vi "Demo Multiple Std Dev Calcs.vi"() -> ()   [LabVIEW 2014, in "Exponential Fit Library.lvlib" / "Fit Exponential.lvclass"]
doc: "This is a simle demonstration of the capabilities of the exponential fit class."
uses:
  Fit Exponential.lvclass
panel:
  out "x-y":u32
  out "XY Graph":cluster{"ChunkSize":i32[], "StdDevOut":dbl[]}(graph)
  in  "ChunkSize":i32[](array[numeric])
  in  "# taus":i32
  in  "tau":dbl=60.0
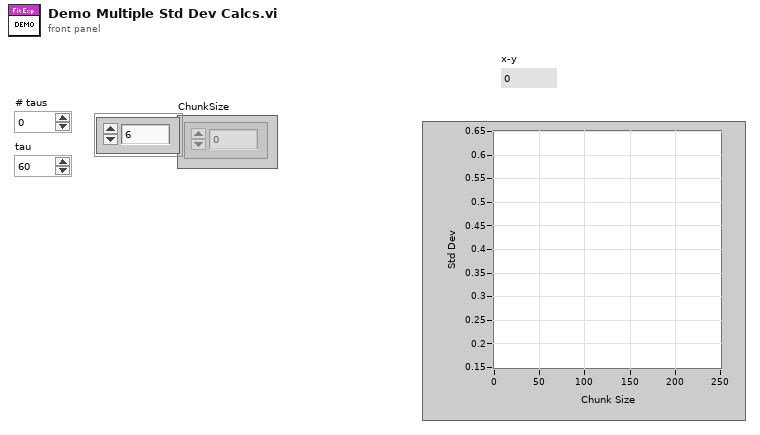
[diagram p1: front panel]
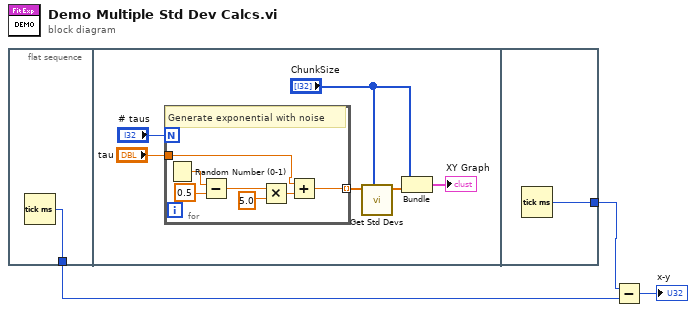
[diagram p0: block diagram]
diagram:
  n1 = flat-sequence {
    tunnel: [w4] -> w2
    tunnel: [w18] -> w3
    frame #0 {
      n2 = Tick Count (ms)() -> (millisecond timer value=w4:u32)
    }
    frame #1 {
      n3 = for {
        N: "# taus" -> [_]
        tunnel: [w12] -> w9 mode=indexing
        tunnel: "tau" -> [w11]
        # "Generate exponential with noise"
        n4 = Random Number (0-1)() -> (number: 0 to 1=w17:dbl)
        n5 = Subtract(x=w17, y=0.5) -> (x-y=w15:dbl)
        n6 = Multiply(x=w15, y=5.0) -> (x*y=w13:dbl)
        n7 = Add(x=w11, y=w13) -> (x+y=w12:dbl)
      }
      n8 = call "Get Std Devs.vi"("ChunkSize"="ChunkSize", "DataIn"=w9) -> ("StdDevOut"=w5:dbl[])  [unwired: 8 in, 1 out]
      n9 = Bundle("ChunkSize"="ChunkSize", "StdDevOut"=w5) -> (→"XY Graph":cluster{"ChunkSize":i32[], "StdDevOut":dbl[]})  [unwired: 1 in]
    }
    frame #2 {
      n10 = Tick Count (ms)() -> (millisecond timer value=w18:u32)
    }
  }
  n11 = Subtract(x=w3, y=w2) -> (x-y=→"x-y":u32)
